vi "Read ADU Packet.vi"(8 "error in":errorcluster, 10 "protocol layer":refnum<class "Network Protocol.lvclass">, 11 "transmission data unit in":refnum<class "Transmission Data Unit.lvclass">) -> (0 "error out":errorcluster, 1 "modbus data unit":refnum<class "Modbus Data Unit.lvclass">, 2 "protocol layer out":refnum<class "Network Protocol.lvclass">, 3 "transmission data unit out":refnum<class "Transmission Data Unit.lvclass">, 5 "PDU Valid?":bool)   [LabVIEW 2013, in "Modbus Library - Advance.lvlib" / "Transmission Data Unit.lvclass"]
doc: "This method reads data off of the chosen bus and attempts to return a modbus modbus data unit in the alotted time."
uses:
  Transmission Data Unit.lvclass
  Modbus Data Unit/Modbus Data Unit.lvclass
  Network Protocol/Network Protocol.lvclass
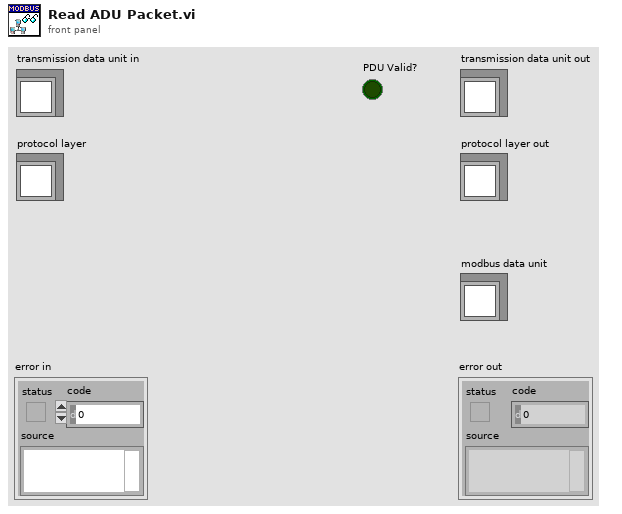
[diagram p1: front panel]
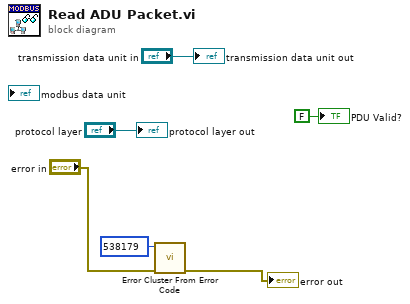
[diagram p0: block diagram]
diagram:
  n1 = call <vilib>:"Error Cluster From Error Code.vi"("error in (no error)"="error in", "error code (0)"=538179) -> ("error out"=→"error out":errorcluster)  [unwired: 7 in]
  "transmission data unit out" <- "transmission data unit in"
  "protocol layer out" <- "protocol layer"
  "PDU Valid?" <- FALSE ("PDU Valid?")
